vi "FPGA.vi"() -> ()   [LabVIEW 2019]
uses:
  <vilib>/rvi/Emulation/niFpgaGetClockAttributes.vi
  <vilib>/rvi/Emulation/niFpgaSctlEmulationGetInTimedLoop.vi
  <vilib>/rvi/Emulation/niFpgaEmulationReportErrorSimple.vi
  <vilib>/rvi/eio/common/nirviEmuTemplateMethod_errors.vi
  <vilib>/rvi/Emulation/niFpgaCriticalErrorInLSC.vi
  <vilib>/eio/EIONode/EIONode.xnode
panel:
  out "LED":i32
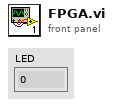
[diagram p1: front panel]
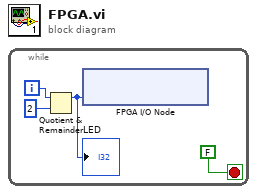
[diagram p0: block diagram]
diagram:
  n1 = while {
    i -> [w4]
    stop <- FALSE stop-if-true
    n2 = Quotient & Remainder(x=w4, y=2) -> (x-y*floor(x/y)=w2:i32)  [unwired: 1 out]
    "LED" <- w2
    n3 = xnode "FPGA I/O Node"("USER FPGA LED"=w2) -> ()  [unwired: 1 in, 1 out]
  }
